vi "fgv_pause.vi"(7 "cmd":enum16{"default", "ini", "pause"}(ring), 8 "error in (no error)":errorcluster caption="error in") -> (0 "error out":errorcluster, 3 "pause":bool)   [LabVIEW 2016]
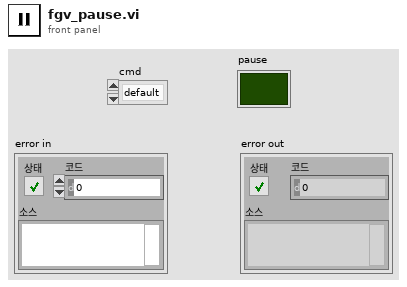
[diagram p1: front panel]
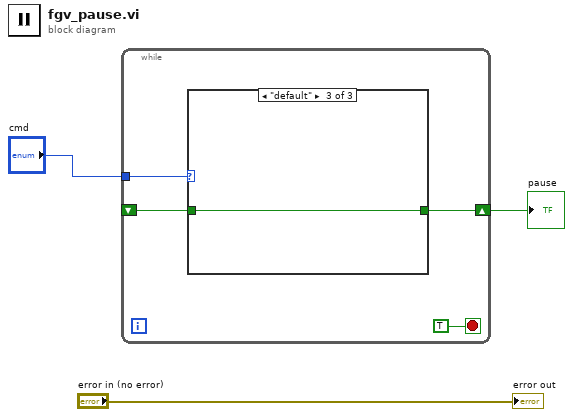
[diagram p0: block diagram]
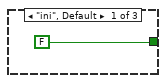
[diagram p2: hidden frame]
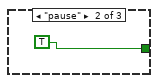
[diagram p3: hidden frame]
diagram:
  n1 = while {
    tunnel: "cmd" -> [w7]
    shift-right: [w5] -> w2
    shift-left: _ -> [w4]
    stop <- TRUE stop-if-true
    n2 = case shown="\"default\"" w7 {
      tunnel: [FALSE TRUE w10] -> w5
      tunnel: w4 -> [_ _ w10]
      frame "ini", Default {
      }
      frame "pause" {
      }
      frame "default" {
      }
    }
  }
  "pause" <- w2
  "error out" <- "error in (no error)"
